vi "Ej6.vi"() -> ()   [LabVIEW 2023]
uses:
  <vilib>/Analysis/baseanly.llb/Mean (DBL).vi
  <vilib>/Analysis/NI_AALBase.lvlib
panel:
  out "mean":dbl format="%#_13g"
  out "min":dbl format="%#_13g"
  out "max":dbl format="%#_13g"
  in  "stop":bool
  out "Current data point":i32
  out "Thermometer":dbl(slide) scale=0.0..100.0
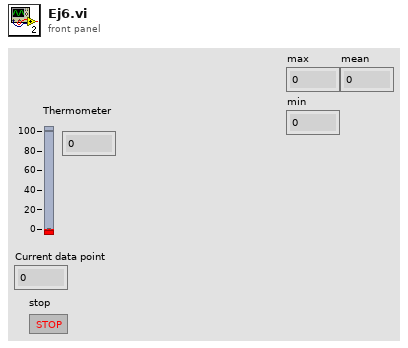
[diagram p1: front panel]
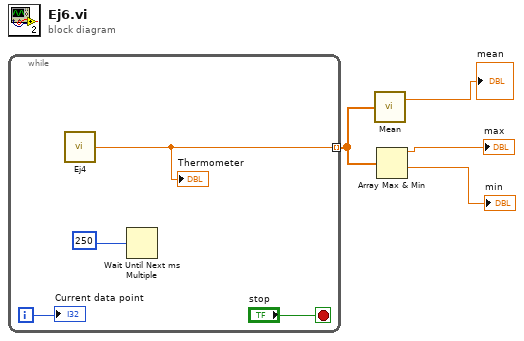
[diagram p0: block diagram]
diagram:
  n1 = while {
    tunnel: [w5] -> w1 mode=indexing
    i -> [w8]
    stop <- "stop" stop-if-true
    n2 = call "Ej4.vi"() -> ("Thermometer"=w5:dbl)  [unwired: 1 in]
    "Thermometer" <- w5
    n3 = Wait Until Next ms Multiple(millisecond multiple=250) -> ()  [unwired: 1 out]
    "Current data point" <- w8
  }
  n4 = call-poly <vilib>:"Mean.vi"("X"=w1) -> ("mean"=→"mean":dbl)  [unwired: 1 out]
  n5 = Array Max & Min(array=w1) -> (max value=→"max":dbl, min value=→"min":dbl)  [unwired: 2 out]
